vi "test21-LosslessRegisterStateMultipleTimesNonCSM.vi"(8 "error in (no error)":errorcluster, 11 "TestCase in":refnum<class "testcase-CSMBroadcast.lvclass">) -> (0 "error out":errorcluster, 3 "TestCase out":refnum<class "testcase-CSMBroadcast.lvclass">)   [LabVIEW 2017, in "testcase-CSMBroadcast.lvclass"]
uses:
  testcase-CSMBroadcast.lvclass
  <vilib>/addons/_JKI Toolkits/VI Tester/TestCase.llb/TestCase.lvclass
  src/user.lib/_NEVSTOP/Communicable State Machine(CSM)/Communicable State Machine.lvlib
  CSM/CSM-Testcase.lvlib
  C:/Program Files (x86)/National Instruments/LabVIEW 2017/vi.lib/addons/_JKI Toolkits/VI Tester/TestCase.llb/TestCase.lvclass
panel:
  out "Arguments":string
  out "ModuleName":string
  out "LoopCount":i32
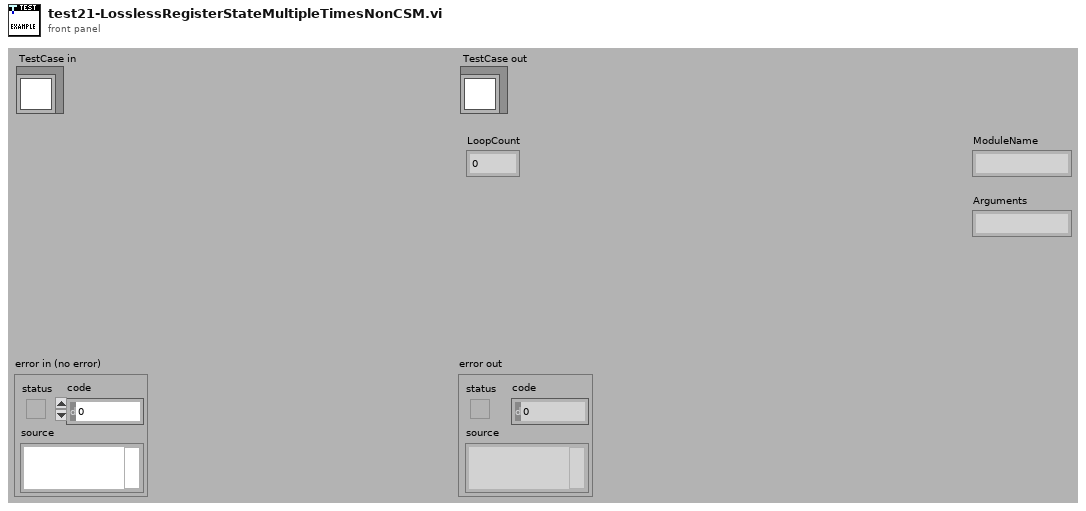
[diagram p1: front panel]
types:
  T1 = cluster{"ModuleName":string, "Status":string, "Arguments":string}
  T2 = cluster{"cluster":cluster{"ModuleName":string, "Status":string, "Arguments":string}, "Counter":u32}
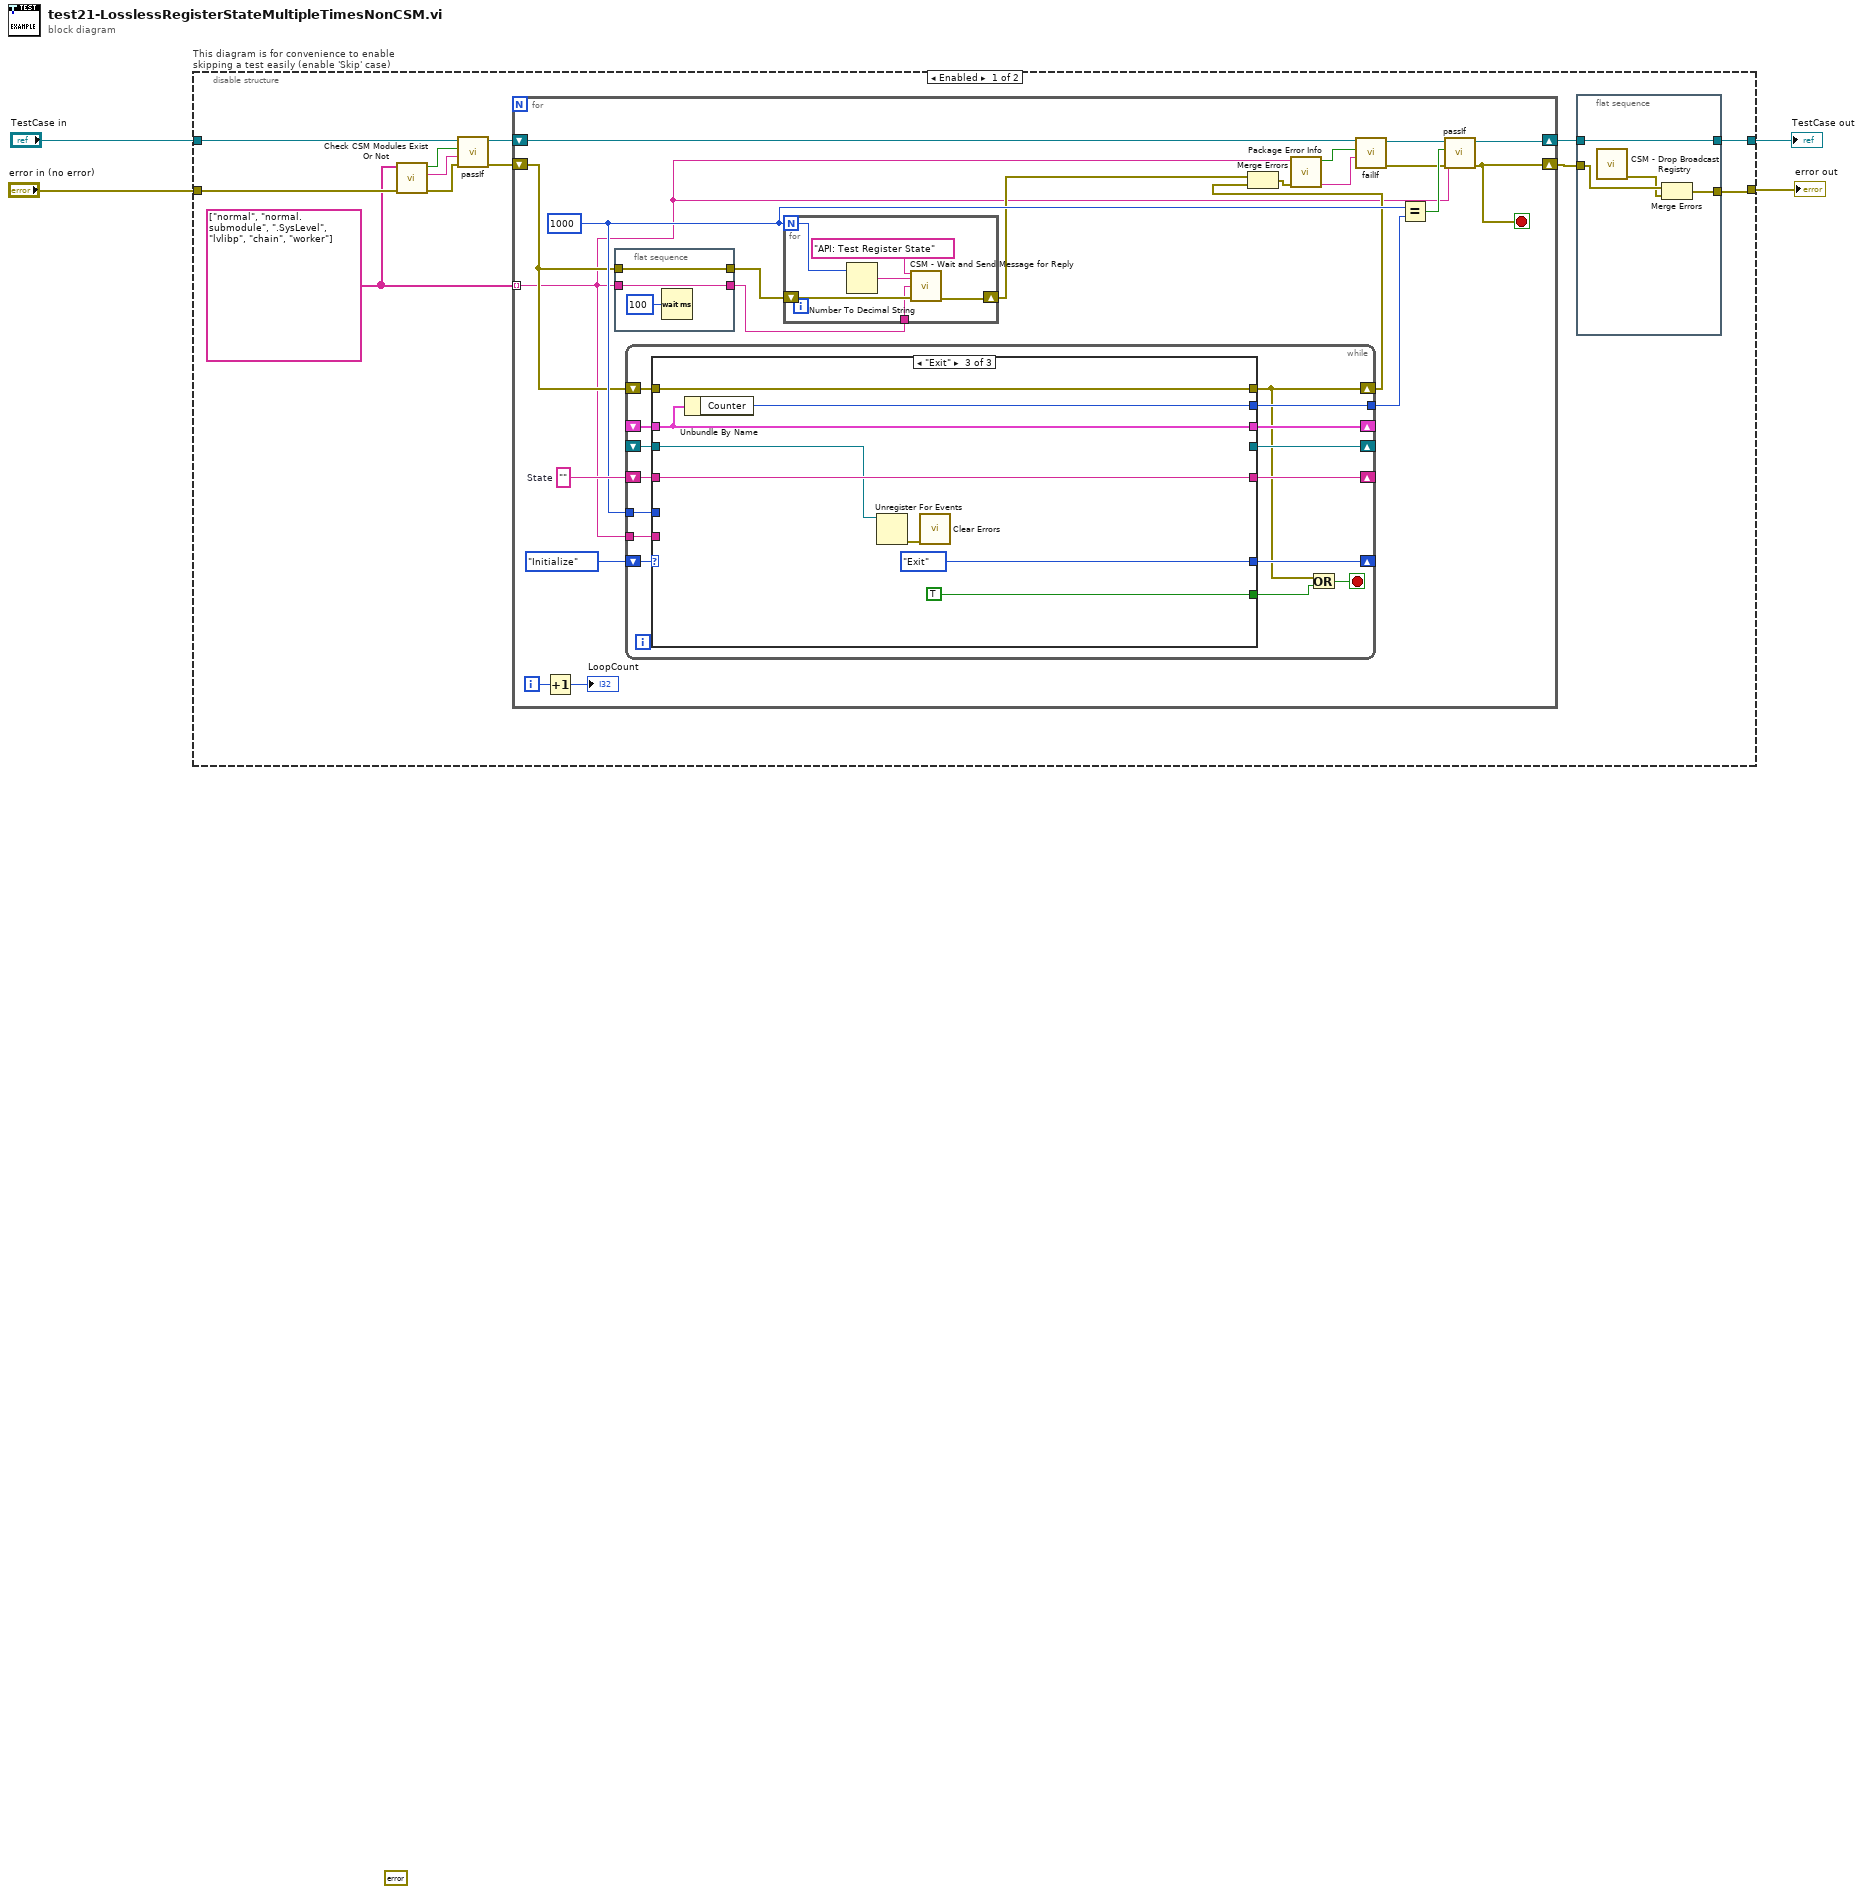
[diagram p0: block diagram]
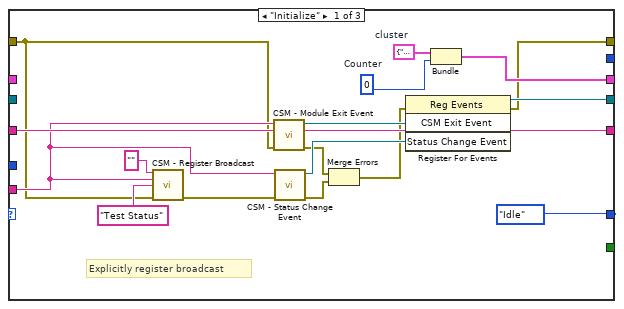
[diagram p2: hidden frame]
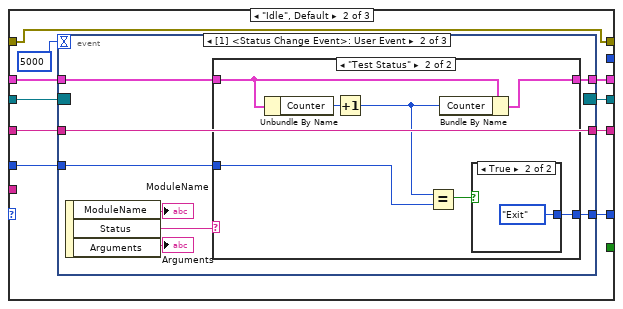
[diagram p3: hidden frame]
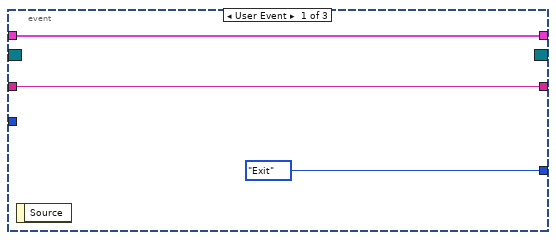
[diagram p4: hidden frame]
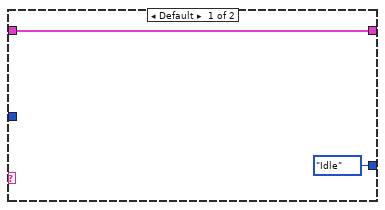
[diagram p5: hidden frame]
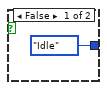
[diagram p6: hidden frame]
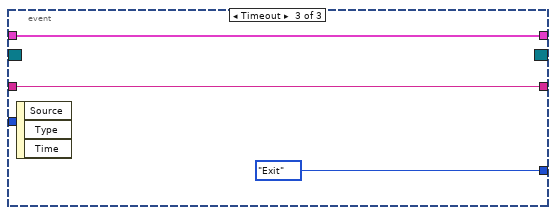
[diagram p7: hidden frame]
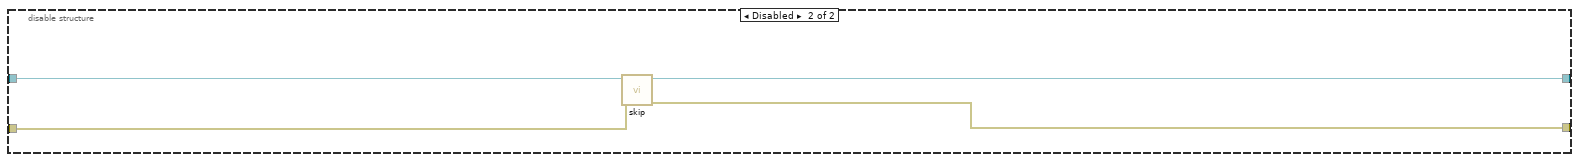
[diagram p8: hidden frame]
diagram:
  (unwired) errorcluster {"status"=FALSE, "code"=0, "source"=""} ("error out")
  n1 = disable-structure "This diagram is for convenience to enable skipping a test easily (enable 'Skip' case)" shown="Enabled" {
    disable-tunnel: "TestCase in" -> [w11 w129]
    disable-tunnel: [w5 w127] -> w2
    disable-tunnel: [w15 w128] -> w1
    disable-tunnel: "error in (no error)" -> [w8 w126]
    frame Enabled {
      w7 = string[] ["normal", "normal.submodule", ".SysLevel", "lvlibp", "chain", "worker"]
      n2 = call "Check CSM Modules Exist Or Not.vi"("error in"=w8, "CSM names in"=w7) -> ("error out"=w12:errorcluster, "Debug string"=w13:string, "All Modules Exist?"=w14:bool)  [unwired: 7 in]
      n3 = call-dynamic "passIf.vi"("error in (no error)"=w12, "message (\"\")"=w13, "pass"=w14, "TestCase in"=w11) -> ("error out"=w9:errorcluster, "TestCase out"=w10:refnum<class "testcase-CSMBroadcast.lvclass">)  [unwired: 6 in]
      n4 = for {
        shift-right: [w39] -> w6
        shift-left: w10 -> [w23]
        shift-right: [w36] -> w16
        shift-left: w9 -> [w30]
        tunnel: w7 -> [w24] mode=indexing
        i -> [w38]
        stop <- w36 stop-if-true
        w32 = 1000
        w40 = ""  # State
        n5 = Increment(x=w38) -> (x+1=→"LoopCount":i32)
        n6 = flat-sequence {
          tunnel: w24 -> [w50]
          tunnel: [w50] -> w35
          tunnel: w30 -> [w48]
          tunnel: [w48] -> w31
          frame #0 {
            n7 = Wait (ms)(milliseconds to wait=u32 100) -> ()  [unwired: 1 out]
          }
        }
        n8 = while {
          shift-right: [w64] -> _
          shift-left: enum16{"Idle", "Initialize", "Exit"}."Initialize" -> [w65]
          shift-right: [w62] -> _
          shift-left: w40 -> [w63]
          shift-right: [w61] -> _
          shift-left: _ -> [w60]
          shift-right: [w59] -> _
          shift-left: _ -> [w58]
          tunnel: w24 -> [w57]
          tunnel: [w56] -> w34
          tunnel: w32 -> [w55]
          shift-right: [w53] -> w27
          shift-left: w30 -> [w54]
          stop <- w51 stop-if-true
          n9 = case shown="\"Exit\"" w65 {
            tunnel: [enum16{"Idle", "Initialize", "Exit"}."Idle" w92 enum16{"Idle", "Initialize", "Exit"}."Exit"] -> w64
            tunnel: [_ _ TRUE] -> w52
            tunnel: w63 -> [w81 w90 w123]
            tunnel: [w81 w91 w123] -> w62
            tunnel: [w79 w88 _] -> w61
            tunnel: w60 -> [_ w89 w122]
            tunnel: [w78 w86 w119] -> w59
            tunnel: w58 -> [_ w87 w119]
            tunnel: w57 -> [w70 _ _]
            tunnel: [_ _ w120] -> w56
            tunnel: w55 -> [_ w84 _]
            tunnel: w54 -> [w68 w83 w118]
            tunnel: [w66 w83 w118] -> w53
            frame "Initialize" {
              w73 = u32 0  # Counter
              w76 = T1 {"ModuleName"="", "Status"="", "Arguments"=""}  # cluster
              # "Explicitly register broadcast"
              n10 = call "CSM - Register Broadcast.vi"("CSM Name(Empty for Broadcast Event)"="", "Source CSM Name (* as Default)"=w70, "Trigger"="Test Status" ("State"), "Error In"=w68) -> ("error out"=w69:errorcluster)  [unwired: 10 in, 1 out]
              n11 = call "CSM - Module Exit Event.vi"("Error In"=w68, "Name (\"\" to Use UUID) In"=w70) -> ("error out"=w75:errorcluster, "CSM Exit Event"=w80:refnum<user-event>)  [unwired: 7 in, 1 out]
              n12 = call "CSM - Status Change Event.vi"("Error In"=w69, "CSM Module"=w70) -> ("error out"=w74:errorcluster, "Status Change Event"=w77:refnum<user-event>)  [unwired: 7 in, 1 out]
              n13 = Merge Errors(w75, w74) -> (w67:errorcluster)
              n14 = register-events(error in=w67, w80, w77) -> (reference out=w79:refnum<event-registration>, error out=w66:errorcluster)  [unwired: 1 in]
              n15 = Bundle("cluster"=w76, "Counter"=w73) -> (w78:T2)  [unwired: 1 in]
            }
            frame "Idle", Default {
              n16 = event shown="[1] <Status Change Event>: User Event" {
                selector: w89 -> [_ _ _]
                dyn-events: [_ _ _] -> w88
                timeout: 5000 -> [_ _ _]
                tunnel: [enum16{"Idle", "Initialize", "Exit"}."Exit" w102 enum16{"Idle", "Initialize", "Exit"}."Exit"] -> w92
                tunnel: w90 -> [w95 w103 w117]
                tunnel: [w95 w103 w117] -> w91
                tunnel: w87 -> [w93 w100 w116]
                tunnel: [w93 w101 w116] -> w86
                tunnel: w84 -> [_ w99 _]
                event User Event {
                  n17 = event-data() -> ()  [unwired: 1 in, 1 out]
                }
                event User Event {
                  n18 = event-data() -> ("ModuleName"=→"ModuleName":string, "Status"=w98:string, "Arguments"=→"Arguments":string)  [unwired: 1 in]
                  n19 = case shown="\"Test Status\"" w98 {
                    tunnel: [enum16{"Idle", "Initialize", "Exit"}."Idle" w112] -> w102
                    tunnel: [w105 w111] -> w101
                    tunnel: w100 -> [w105 w110]
                    tunnel: w99 -> [_ w106]
                    frame Default {
                    }
                    frame "Test Status" {
                      n20 = Unbundle By Name(w110) -> ("Counter"=w109:u32)
                      n21 = Increment(x=w109) -> (x+1=w107:u32)
                      n22 = Equal?(x=w107, y=w106) -> (x = y?=w108:bool)
                      n23 = Bundle By Name(cluster=w110, "Counter"=w107) -> (w111:T2)
                      n24 = case shown="True" w108 {
                        tunnel: [enum16{"Idle", "Initialize", "Exit"}."Idle" enum16{"Idle", "Initialize", "Exit"}."Exit"] -> w112
                        frame False {
                        }
                        frame True {
                        }
                      }
                    }
                  }
                }
                event Timeout {
                  n25 = event-data() -> ()  [unwired: 1 in, 3 out]
                }
              }
            }
            frame "Exit" {
              n26 = Unbundle By Name(w119) -> ("Counter"=w120:u32)
              n27 = Unregister For Events(event registration refnum=w122) -> (error out=w121:errorcluster)  [unwired: 1 in]
              n28 = call <vilib>:"Clear Errors.vi"("error in (no error)"=w121) -> ()  [unwired: 5 in, 2 out]
            }
          }
          n29 = Or(x=w53, y=w52) -> (x .or. y?=w51:bool)
        }
        n30 = for {
          N: w32 -> [w45]
          shift-right: [w43] -> w25
          shift-left: w31 -> [w44]
          tunnel: w35 -> [w42]
          n31 = Number To Decimal String(number=w45) -> (decimal integer string=w46:string)  [unwired: 1 in]
          n32 = call "CSM - Wait and Send Message for Reply.vi"("State"="API: Test Register State", "Arguments (\"\")"=w46, "Target Module"=w42, "Error In (No Error)"=w44) -> ("error out"=w43:errorcluster)  [unwired: 8 in, 3 out]
        }
        n33 = Merge Errors(w25, w27) -> (w26:errorcluster)
        n34 = call "Package Error Info.vi"("error in"=w26, "String in"=w24) -> ("packed error info out"=w28:string, "error status"=w29:bool)  [unwired: 8 in]
        n35 = call-dynamic "failIf.vi"("message (\"\")"=w28, "fail"=w29, "TestCase in"=w23) -> ("error out"=w21:errorcluster, "TestCase out"=w22:refnum<class "testcase-CSMBroadcast.lvclass">)  [unwired: 7 in]
        n36 = Equal?(x=w32, y=w34) -> (x = y?=w33:bool)
        n37 = call-dynamic "passIf.vi"("error in (no error)"=w21, "message (\"\")"=w24, "pass"=w33, "TestCase in"=w22) -> ("error out"=w36:errorcluster, "TestCase out"=w39:refnum<class "testcase-CSMBroadcast.lvclass">)  [unwired: 6 in]
      }
      n38 = flat-sequence {
        tunnel: w16 -> [w20]
        tunnel: [w19] -> w15
        tunnel: w6 -> [w17]
        tunnel: [w17] -> w5
        frame #0 {
          n39 = call "CSM - Drop Broadcast Registry.vi"() -> ("error out"=w18:errorcluster)  [unwired: 15 in]
          n40 = Merge Errors(w20, w18) -> (w19:errorcluster)
        }
      }
    }
    frame Disabled {
      # "skip test result while test is under development"
      n41 = call <vilib>:"skip.vi"("error in (no error)"=w126, "TestCase in"=w129) -> ("error out"=w128:errorcluster, "TestCase out"=w127:refnum<class "testcase-CSMBroadcast.lvclass">)  [unwired: 8 in]
    }
  }
  "error out" <- w1
  "TestCase out" <- w2
